vi "FGV.vi"(7 "FGV State":T1, 8 "error in (no error)":errorcluster, 11 "Path In":path) -> (0 "error out":errorcluster, 3 "Path Out":path)   [LabVIEW 2021, in "Path Utilities.lvlib"]
uses:
  Path Utilities.lvlib
  TypeDefs/FGV State.ctl
  TypeDefs/FGV Data.ctl
  <vilib>/Utility/sysdir.llb/System Directory Type.ctl
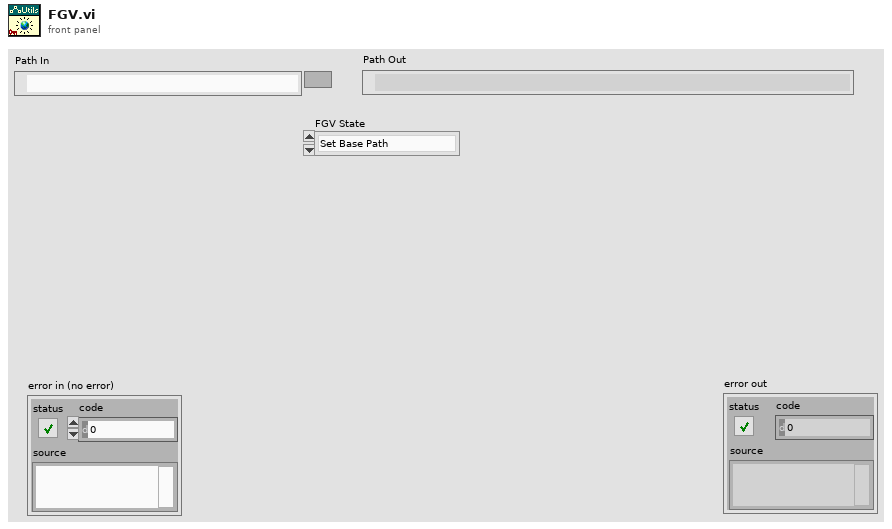
[diagram p1: front panel]
types:
  T1 = typedef "Path Utilities.lvlib/FGV State.ctl" = enum16{"Set Base Path", "Get Program Files", "Get Program Data", "Get App Data Local", "Get App Data Roaming", "Get User Documents", "Get Public Documents"}
  T2 = typedef "Path Utilities.lvlib/FGV Data.ctl" = cluster{"Base Path":path}
  T3 = typedef "System Directory Type.ctl" = i32
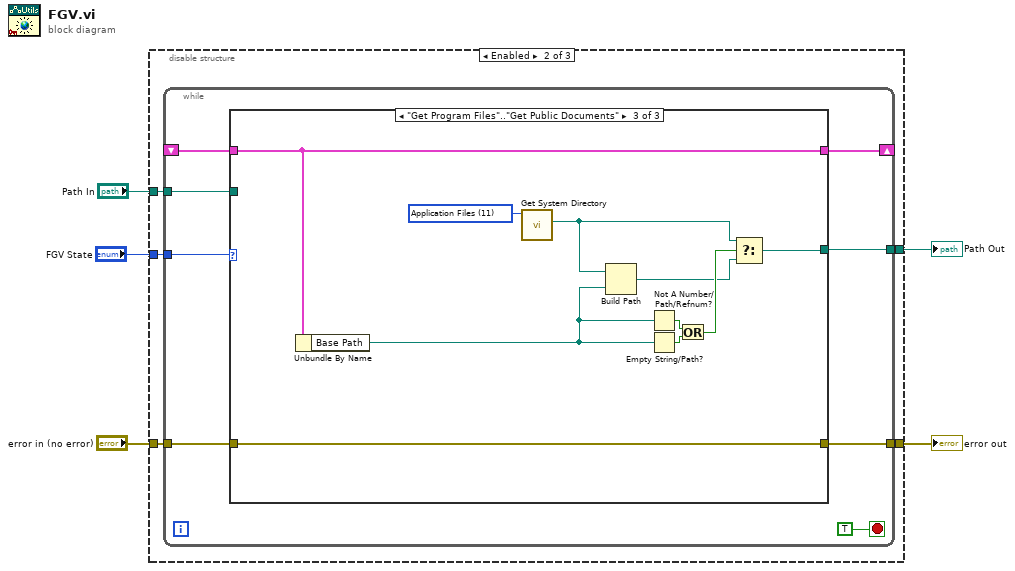
[diagram p0: block diagram]
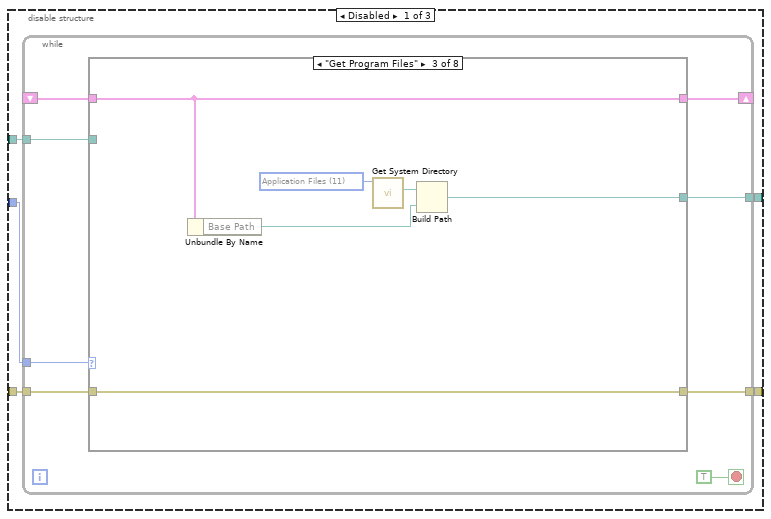
[diagram p2: hidden frame]
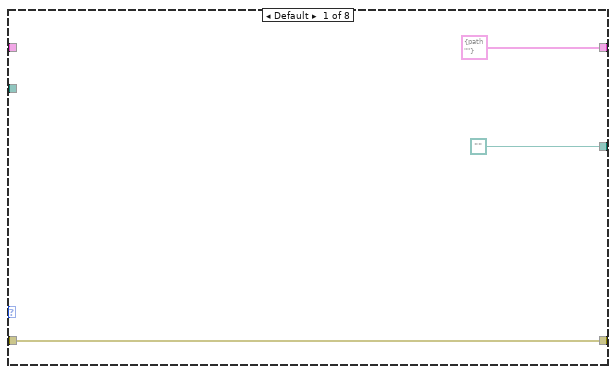
[diagram p3: hidden frame]
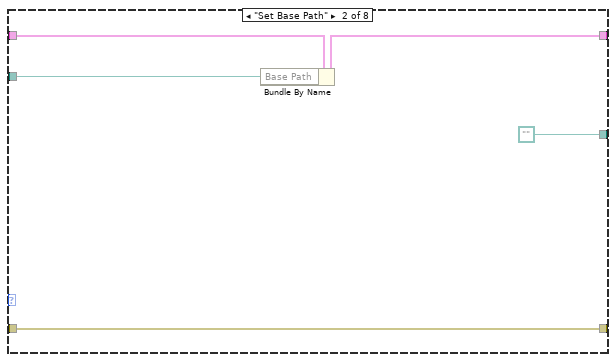
[diagram p4: hidden frame]
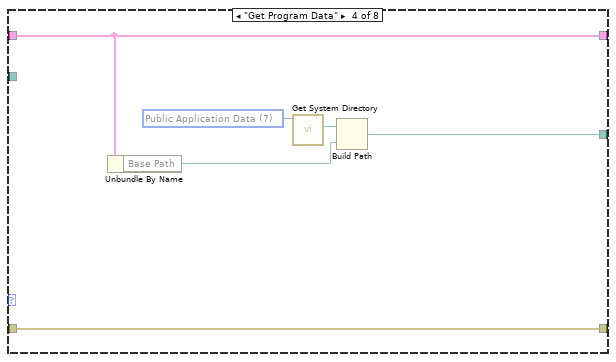
[diagram p5: hidden frame]
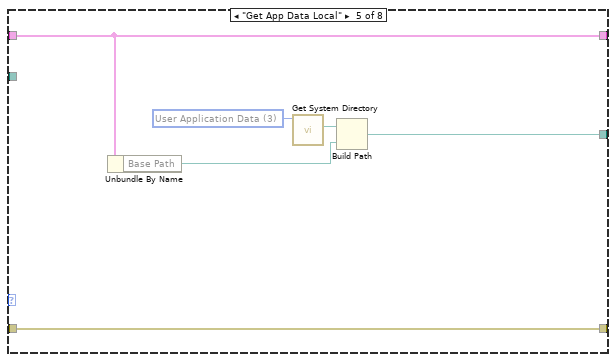
[diagram p6: hidden frame]
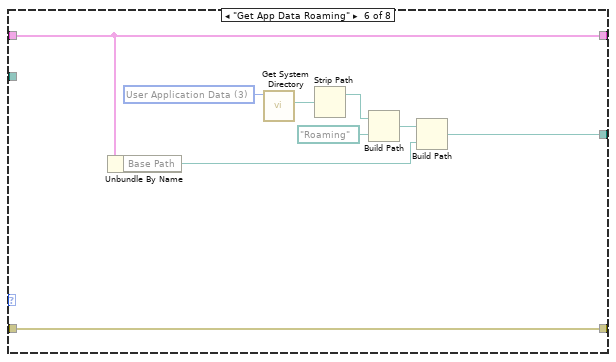
[diagram p7: hidden frame]
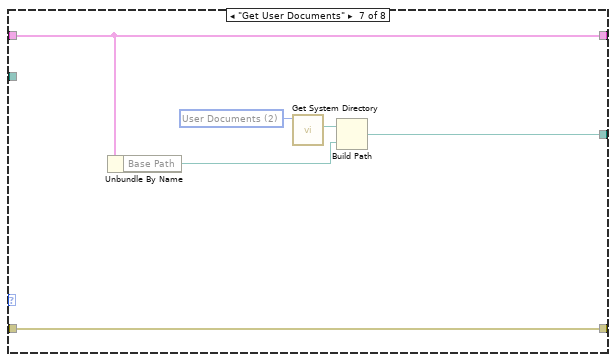
[diagram p8: hidden frame]
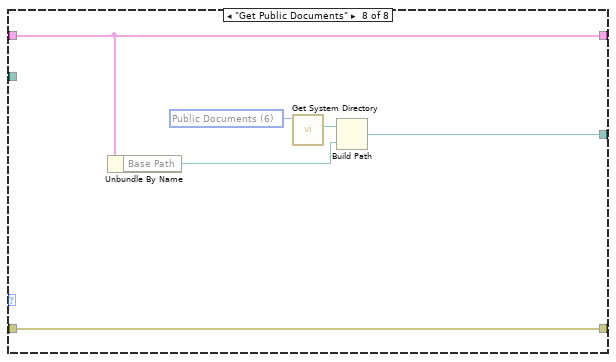
[diagram p9: hidden frame]
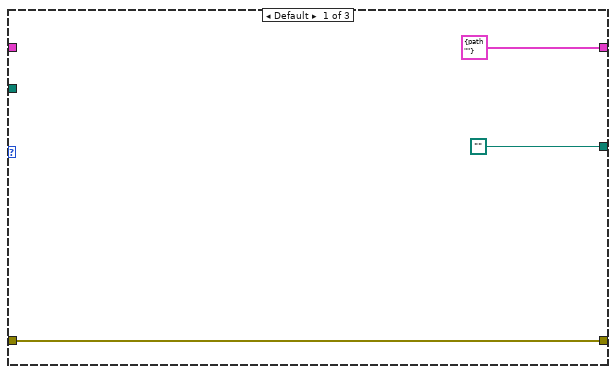
[diagram p10: hidden frame]
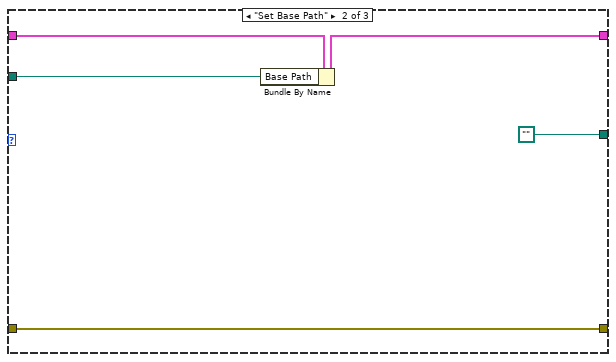
[diagram p11: hidden frame]
diagram:
  n1 = disable-structure shown="Enabled" {
    disable-tunnel: "FGV State" -> [w10 w70 _]
    disable-tunnel: "error in (no error)" -> [w9 w69 _]
    disable-tunnel: [w8 w68 _] -> w3
    disable-tunnel: "Path In" -> [w7 w67 _]
    disable-tunnel: [w6 w66 _] -> w1
    frame Disabled {
      n2 = while {
        shift-right: [w14] -> _
        shift-left: _ -> [w12]
        tunnel: w10 -> [w17]
        tunnel: w9 -> [w16]
        tunnel: [w15] -> w8
        tunnel: w7 -> [w13]
        tunnel: [w11] -> w6
        stop <- TRUE stop-if-true
        n3 = case shown="\"Get Program Files\"" w17 {
          tunnel: w16 -> [w20 w26 w27 w33 w39 w49 w54 w60]
          tunnel: [w20 w26 w27 w33 w39 w49 w54 w60] -> w15
          tunnel: [T2 {"Base Path"=path ""} ("FGV Data") w25 w31 w37 w43 w52 w58 w64] -> w14
          tunnel: w13 -> [_ w24 _ _ _ _ _ _]
          tunnel: w12 -> [_ w23 w31 w37 w43 w52 w58 w64]
          tunnel: [path "" path "" w28 w34 w40 w50 w55 w61] -> w11
          frame Default {
          }
          frame "Set Base Path" {
            n4 = Bundle By Name(cluster=w23, "Base Path"=w24) -> (w25:T2)
          }
          frame "Get Program Files" {
            w32 = T3 11 items=["User Home"=0, "User Desktop"=1, "User Documents"=2, "User Application Data"=3, "User Preferences"=4, "User Temporary"=5, "Public Documents"=6, "Public Application Data"=7, "Public Preferences"=8, "Public Cache"=13, "System Core Libraries"=9, "System Installed Libraries"=10, "Application Files"=11, "Boot Volume Root"=12] ("system directory type")
            n5 = Unbundle By Name(w31) -> ("Base Path"=w29:path)
            n6 = call <vilib>:"Get System Directory.vi"("system directory type"=w32) -> ("system directory"=w30:path)  [unwired: 10 in]
            n7 = Build Path(base path=w30, name or relative path=w29) -> (appended path=w28:path)
          }
          frame "Get Program Data" {
            w38 = T3 7 items=["User Home"=0, "User Desktop"=1, "User Documents"=2, "User Application Data"=3, "User Preferences"=4, "User Temporary"=5, "Public Documents"=6, "Public Application Data"=7, "Public Preferences"=8, "Public Cache"=13, "System Core Libraries"=9, "System Installed Libraries"=10, "Application Files"=11, "Boot Volume Root"=12] ("system directory type")
            n8 = Unbundle By Name(w37) -> ("Base Path"=w35:path)
            n9 = call <vilib>:"Get System Directory.vi"("system directory type"=w38) -> ("system directory"=w36:path)  [unwired: 10 in]
            n10 = Build Path(base path=w36, name or relative path=w35) -> (appended path=w34:path)
          }
          frame "Get App Data Local" {
            w44 = T3 3 items=["User Home"=0, "User Desktop"=1, "User Documents"=2, "User Application Data"=3, "User Preferences"=4, "User Temporary"=5, "Public Documents"=6, "Public Application Data"=7, "Public Preferences"=8, "Public Cache"=13, "System Core Libraries"=9, "System Installed Libraries"=10, "Application Files"=11, "Boot Volume Root"=12] ("system directory type")
            n11 = Unbundle By Name(w43) -> ("Base Path"=w41:path)
            n12 = call <vilib>:"Get System Directory.vi"("system directory type"=w44) -> ("system directory"=w42:path)  [unwired: 10 in]
            n13 = Build Path(base path=w42, name or relative path=w41) -> (appended path=w40:path)
          }
          frame "Get App Data Roaming" {
            w53 = T3 3 items=["User Home"=0, "User Desktop"=1, "User Documents"=2, "User Application Data"=3, "User Preferences"=4, "User Temporary"=5, "Public Documents"=6, "Public Application Data"=7, "Public Preferences"=8, "Public Cache"=13, "System Core Libraries"=9, "System Installed Libraries"=10, "Application Files"=11, "Boot Volume Root"=12] ("system directory type")
            n14 = Unbundle By Name(w52) -> ("Base Path"=w51:path)
            n15 = call <vilib>:"Get System Directory.vi"("system directory type"=w53) -> ("system directory"=w48:path)  [unwired: 10 in]
            n16 = Strip Path(path=w48) -> (stripped path=w47:path)  [unwired: 1 out]
            n17 = Build Path(base path=w47, name or relative path=path "Roaming") -> (appended path=w46:path)
            n18 = Build Path(base path=w46, name or relative path=w51) -> (appended path=w50:path)
          }
          frame "Get User Documents" {
            w59 = T3 2 items=["User Home"=0, "User Desktop"=1, "User Documents"=2, "User Application Data"=3, "User Preferences"=4, "User Temporary"=5, "Public Documents"=6, "Public Application Data"=7, "Public Preferences"=8, "Public Cache"=13, "System Core Libraries"=9, "System Installed Libraries"=10, "Application Files"=11, "Boot Volume Root"=12] ("system directory type")
            n19 = Unbundle By Name(w58) -> ("Base Path"=w56:path)
            n20 = call <vilib>:"Get System Directory.vi"("system directory type"=w59) -> ("system directory"=w57:path)  [unwired: 10 in]
            n21 = Build Path(base path=w57, name or relative path=w56) -> (appended path=w55:path)
          }
          frame "Get Public Documents" {
            w65 = T3 6 items=["User Home"=0, "User Desktop"=1, "User Documents"=2, "User Application Data"=3, "User Preferences"=4, "User Temporary"=5, "Public Documents"=6, "Public Application Data"=7, "Public Preferences"=8, "Public Cache"=13, "System Core Libraries"=9, "System Installed Libraries"=10, "Application Files"=11, "Boot Volume Root"=12] ("system directory type")
            n22 = Unbundle By Name(w64) -> ("Base Path"=w62:path)
            n23 = call <vilib>:"Get System Directory.vi"("system directory type"=w65) -> ("system directory"=w63:path)  [unwired: 10 in]
            n24 = Build Path(base path=w63, name or relative path=w62) -> (appended path=w61:path)
          }
        }
      }
    }
    frame Enabled {
      n25 = while {
        shift-right: [w74] -> _
        shift-left: _ -> [w72]
        tunnel: w70 -> [w77]
        tunnel: w69 -> [w76]
        tunnel: [w75] -> w68
        tunnel: w67 -> [w73]
        tunnel: [w71] -> w66
        stop <- TRUE stop-if-true
        n26 = case shown="\"Get Program Files\"..\"Get Public Documents\"" w77 {
          tunnel: w76 -> [w80 w86 w94]
          tunnel: [w80 w86 w94] -> w75
          tunnel: [T2 {"Base Path"=path ""} ("FGV Data") w85 w95] -> w74
          tunnel: w73 -> [_ w84 _]
          tunnel: w72 -> [_ w83 w95]
          tunnel: [path "" path "" w89] -> w71
          frame Default {
          }
          frame "Set Base Path" {
            n27 = Bundle By Name(cluster=w83, "Base Path"=w84) -> (w85:T2)
          }
          frame "Get Program Files".."Get Public Documents" {
            w96 = T3 11 items=["User Home"=0, "User Desktop"=1, "User Documents"=2, "User Application Data"=3, "User Preferences"=4, "User Temporary"=5, "Public Documents"=6, "Public Application Data"=7, "Public Preferences"=8, "Public Cache"=13, "System Core Libraries"=9, "System Installed Libraries"=10, "Application Files"=11, "Boot Volume Root"=12] ("system directory type")
            n28 = Unbundle By Name(w95) -> ("Base Path"=w90:path)
            n29 = call <vilib>:"Get System Directory.vi"("system directory type"=w96) -> ("system directory"=w87:path)  [unwired: 10 in]
            n30 = Build Path(base path=w87, name or relative path=w90) -> (appended path=w88:path)
            n31 = Not A Number/Path/Refnum?(number/path/refnum=w90) -> (NaN/Path/Refnum?=w93:bool)
            n32 = Empty String/Path?(string/path=w90) -> (empty?=w92:bool)
            n33 = Or(x=w93, y=w92) -> (x .or. y?=w91:bool)
            n34 = Select(t=w87, s=w91, f=w88) -> (s? t:f=w89:path)
          }
        }
      }
    }
    frame Disabled {
    }
  }
  "error out" <- w3
  "Path Out" <- w1
